vi "TCP Engine configuration data location.vi"(11 "Directory":path) -> (1 "Serial":path, 2 "DI":path, 3 "DO":path, 4 "AI":path)   [LabVIEW 2024]
panel:
  out "AO":path
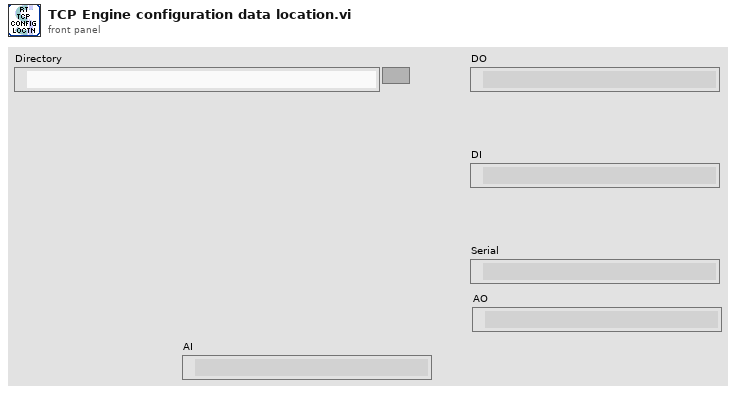
[diagram p1: front panel]
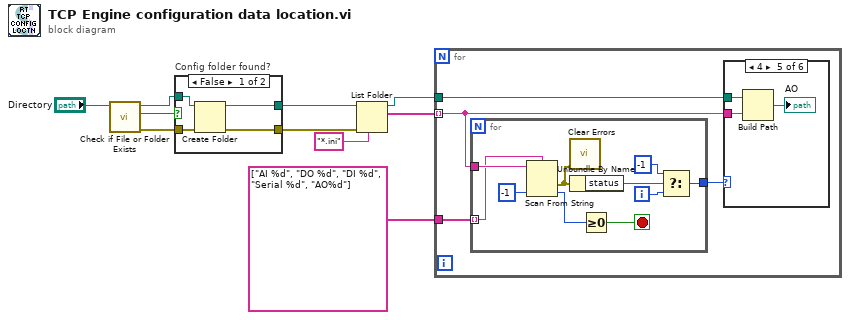
[diagram p0: block diagram]
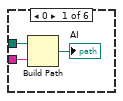
[diagram p2: hidden frame]
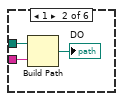
[diagram p3: hidden frame]
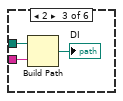
[diagram p4: hidden frame]
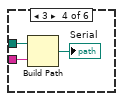
[diagram p5: hidden frame]
diagram:
  n1 = call <vilib>:"Check if File or Folder Exists.vi"("path"="Directory") -> ("error out"=w3:errorcluster, "file or folder exists?"=w1:bool, "dup path"=w2:path)  [unwired: 8 in]
  n2 = case "Config folder found?" shown="False" w1 {
    tunnel: w2 -> [w14 w16]
    tunnel: w3 -> [w13 w15]
    tunnel: [w12 w16] -> w4
    tunnel: [w11 w15] -> w6
    frame False {
      n3 = Create Folder(path (use dialog)=w14, error in=w13) -> (created path=w12:path, error out=w11:errorcluster)  [unwired: 1 in, 1 out]
    }
    frame True {
    }
  }
  n4 = List Folder(path=w4, pattern="*.ini", error in=w6) -> (path out=w10:path, filenames=w8:string[])  [unwired: 1 in, 2 out]
  n5 = for {
    tunnel: w8 -> [w19] mode=indexing
    tunnel: string[] ["AI %d", "DO %d", "DI %d", "Serial %d", "AO%d"] -> [w18]
    tunnel: w10 -> [w20]
    n6 = for {
      tunnel: [w23] -> w17
      tunnel: w19 -> [w29]
      tunnel: w18 -> [w28] mode=indexing
      i -> [w26]
      stop <- w25 stop-if-true
      n7 = Scan From String(format string=w28, input string=w29, default 1=-1 ("default value 1")) -> (error out=w24:errorcluster, output 1=w27:i32)  [unwired: 2 in, 2 out]
      n8 = call <vilib>:"Clear Errors.vi"("error in (no error)"=w24) -> ()  [unwired: 5 in, 2 out]
      n9 = Unbundle By Name(w24) -> ("status"=w21:bool)
      n10 = Greater Or Equal To 0?(x=w27) -> (x >= 0?=w25:bool)
      n11 = Select(t=-1, s=w21, f=w26) -> (s? t:f=w23:i32)
    }
    n12 = case shown="4" w17 {
      tunnel: w20 -> [w33 w36 w39 w42 w45 _]
      tunnel: w19 -> [w32 w35 w38 w41 w44 _]
      frame 0 {
        n13 = Build Path(base path=w33, name or relative path=w32) -> (appended path=→"AI":path)
      }
      frame 1 {
        n14 = Build Path(base path=w36, name or relative path=w35) -> (appended path=→"DO":path)
      }
      frame 2 {
        n15 = Build Path(base path=w39, name or relative path=w38) -> (appended path=→"DI":path)
      }
      frame 3 {
        n16 = Build Path(base path=w42, name or relative path=w41) -> (appended path=→"Serial":path)
      }
      frame 4 {
        n17 = Build Path(base path=w45, name or relative path=w44) -> (appended path=→"AO":path)
      }
      frame -1, Default {
      }
    }
  }
